vi "cm2nm_transform_reference_location.vi"(0 "Sample locations of Interest":refnum<vi>, 1 "Sample_Information":T3, 2 "TransformReferenceSessionIndex":i32, 3 "A - Transformation Matrix":T1, 4 "Enter New Point IN":T2, 5 "C":T1, 7 "B - vector offset":T1, 8 "TopLevelDataFilePath":path) -> (6 "Enter New Point OUT":T2)   [LabVIEW 2011]
doc: "From selected spot on the session vs spot table on the top level GUI perform the transformatio for the current session."
uses:
  <vilib>/Analysis/Matrix/Datatypes/RealMatrix.ctl
  cm2nm_coordinate_information_v2.ctl
  <vilib>/Analysis/Matrix/NI_Matrix.lvlib
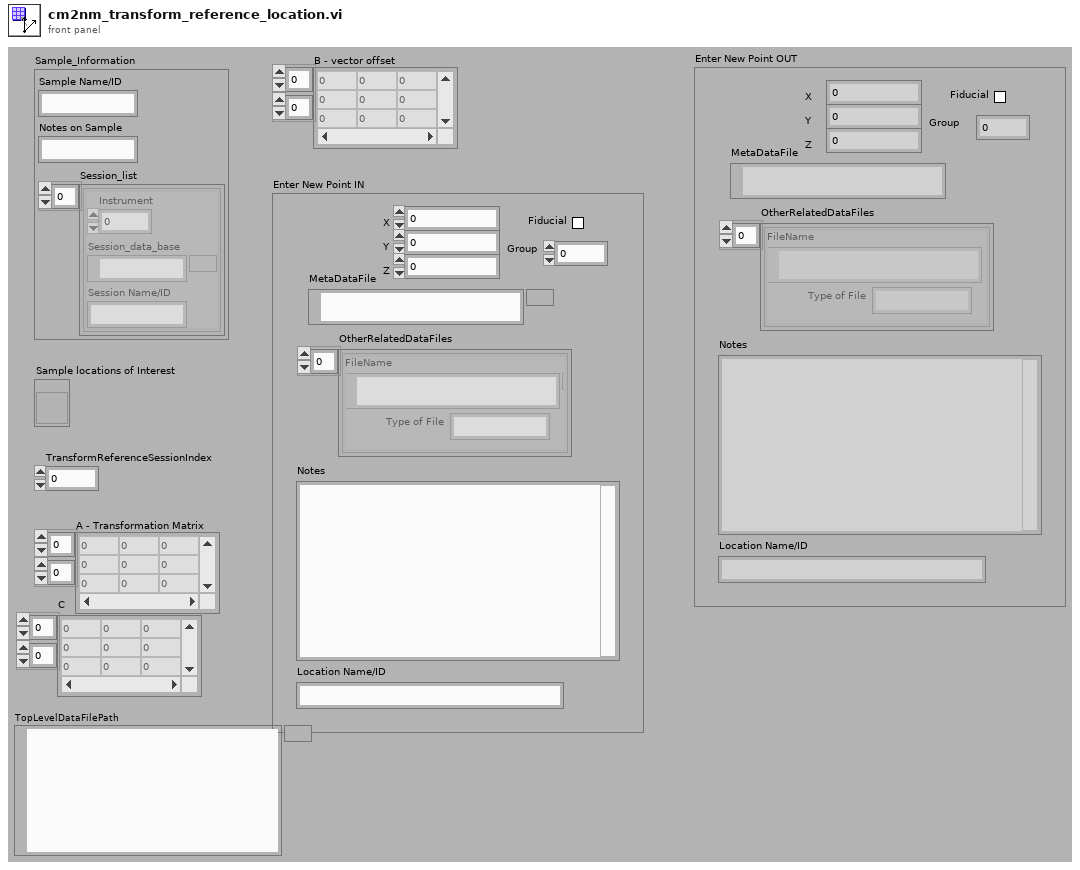
[diagram p1: front panel]
types:
  T1 = typedef "NI_Matrix.lvlib/RealMatrix.ctl" = dbl[][]
  T2 = typedef "cm2nm_coordinate_information_v2.ctl" = cluster{"MetaDataFile":path, "X":dbl, "Y":dbl, "Z":dbl, "Group":i32, "Rotation":dbl[unit], "Fiducial":bool, "Magnification":dbl, "Working_Distance":dbl, "Notes":string, "Location Name/ID":string, "OtherRelatedDataFiles":cluster{"Type of File":string, "FileName":path}[], "Available":bool}
  T3 = cluster{"Sample Name/ID":string, "Notes on Sample":string, "Session_list":cluster{"Instrument":u16, "Session_data_base":path, "Session Name/ID":string}[]}
  T4 = typedef "LVRowAndColumnTypeDef.ctl" = cluster{"Row":i32, "Column":i32}
  T5 = cluster{"Instrument":u16, "Session_data_base":path, "Session Name/ID":string}[]
  T6 = cluster{"Instrument":u16, "Session_data_base":path, "Session Name/ID":string}
  T7 = typedef "cm2nm_sample_set.ctl" = cluster{"CollectionOfPoints":T2[], "Instrument":T8, "CollectionFile":path, "Session Name/ID":string, "SessionNotes":string}
  T8 = typedef "Instrument_type_enum_v2.ctl" = enum16{"Unknown", "Philips FEI SEM IRC", "JEOL 7000F EML_MFC", "MXRD MFC", "JEOL_EPMA"}
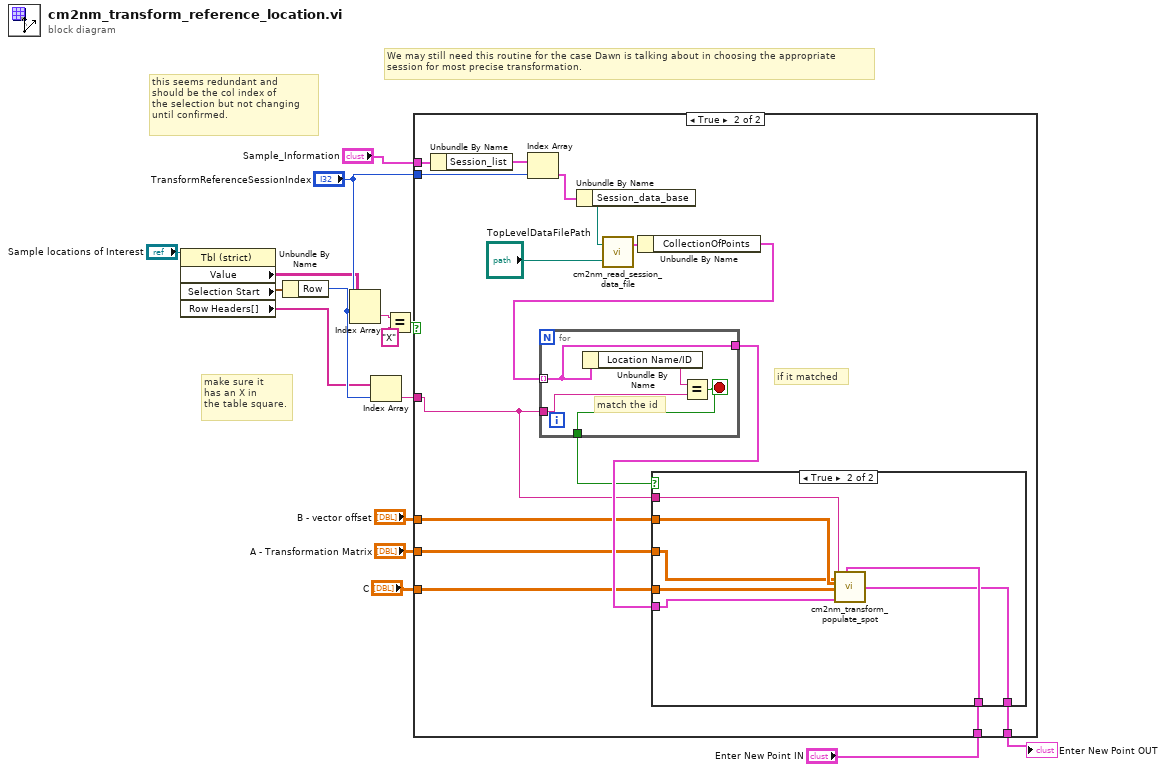
[diagram p0: block diagram]
diagram:
  # "We may still need this routine for the case Dawn is talking about in choosing the appropriate\nsession for most precise transformation."
  # "make sure it\nhas an X in\nthe table square."
  # "this seems redundant and\nshould be the col index of\nthe selection but not changing \nuntil confirmed."
  n1 = property class="Tbl (strict)"(reference="Sample locations of Interest") -> ("Value"=w3:string[][], "Selection Start"=w4:T4, "Row Headers[]"=w8:string[])  [unwired: 1 in, 2 out]
  n2 = Unbundle By Name(w4) -> ("Row"=w9:i32)
  n3 = Index Array(array=w3, index (row)=w9, index (col)="TransformReferenceSessionIndex") -> (element=w6:string)
  n4 = Index Array(array=w8, index=w9) -> (element=w10:string)
  n5 = Equal?(x=w6, y="X") -> (x = y?=w14:bool)
  n6 = case shown="True" w14 {
    tunnel: "TransformReferenceSessionIndex" -> [_ w32]
    tunnel: w10 -> [_ w25]
    tunnel: "Enter New Point IN" -> [w17 w24]
    tunnel: "Sample_Information" -> [_ w23]
    tunnel: [w17 w22] -> w13
    tunnel: "B - vector offset" -> [_ w21]
    tunnel: "A - Transformation Matrix" -> [_ w20]
    tunnel: "C" -> [_ w18]
    frame False {
    }
    frame True {
      # "if it matched"
      n7 = Unbundle By Name(w23) -> ("Session_list"=w33:T5)
      n8 = Index Array(array=w33, index=w32) -> (element=w31:T6)
      n9 = Unbundle By Name(w31) -> ("Session_data_base"=w30:path)
      n10 = call "cm2nm_read_session_data_file.vi"("TopLevelDataFilePath"="TopLevelDataFilePath", "Session_data_base"=w30) -> ("Session Information"=w29:T7)  [unwired: 1 in]
      n11 = Unbundle By Name(w29) -> ("CollectionOfPoints"=w28:T2[])
      n12 = for {
        tunnel: w28 -> [w43] mode=indexing
        tunnel: w25 -> [w44]
        tunnel: [w43] -> w27
        tunnel: [w42] -> w26
        stop <- w42 stop-if-true
        # "match the id"
        n13 = Unbundle By Name(w43) -> ("Location Name/ID"=w45:string)
        n14 = Equal?(x=w45, y=w44) -> (x = y?=w42:bool)
      }
      n15 = case shown="True" w26 {
        tunnel: w27 -> [_ w41]
        tunnel: w25 -> [_ w36]
        tunnel: w24 -> [w34 w40]
        tunnel: [w34 w39] -> w22
        tunnel: w21 -> [_ w38]
        tunnel: w20 -> [_ w37]
        tunnel: w18 -> [_ w35]
        frame False {
        }
        frame True {
          n16 = call "cm2nm_transform_populate_spot.vi"("NewPointIn"=w40, "A - Transformation Matrix"=w37, "Previous Session Spot"=w41, "C"=w35, "B - vector offset"=w38, "Spot_ID"=w36) -> ("NewPointOut"=w39:T2)
        }
      }
    }
  }
  "Enter New Point OUT" <- w13
